vi "WaitForExp.vi"(8 "error in (no error)":errorcluster, 10 "expression":string, 11 "Server":path) -> (0 "error out":errorcluster, 2 "REPL":string)   [LabVIEW 2020]
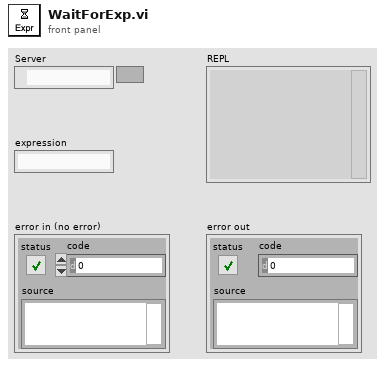
[diagram p1: front panel]
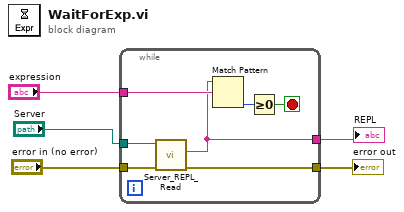
[diagram p0: block diagram]
diagram:
  n1 = while {
    tunnel: "error in (no error)" -> [w12]
    tunnel: "Server" -> [w11]
    tunnel: [w8] -> w4
    tunnel: "expression" -> [w7]
    tunnel: [w6] -> w1
    stop <- w9 stop-if-true
    n2 = call "Server_REPL_Read.vi"("error in (no error)"=w12, "Server"=w11) -> ("error out"=w8:errorcluster, "REPL"=w6:string)  [unwired: 7 in, 1 out]
    n3 = Match Pattern(string=w6, regular expression=w7) -> (offset past match=w10:i32)  [unwired: 1 in, 3 out]
    n4 = Greater Or Equal To 0?(x=w10) -> (x >= 0?=w9:bool)
  }
  "error out" <- w4
  "REPL" <- w1
